vi "Main.vi"() -> ()   [LabVIEW 2016]
uses:
  Code/MainFGV/FGV_mods.ctl
  Code/TypeDefs/specimen_info.ctl
  <vilib>/Analysis/baseanly.llb/Mean (DBL).vi
  <vilib>/Analysis/NI_AALBase.lvlib
panel:
  out "Resultados":string[][](table)
  out "plot":cluster{"strain":dbl[], "stress":dbl[]}[](graph) caption="XY Graph"
  in  "test_file":path caption="Arquivo do ensaio"
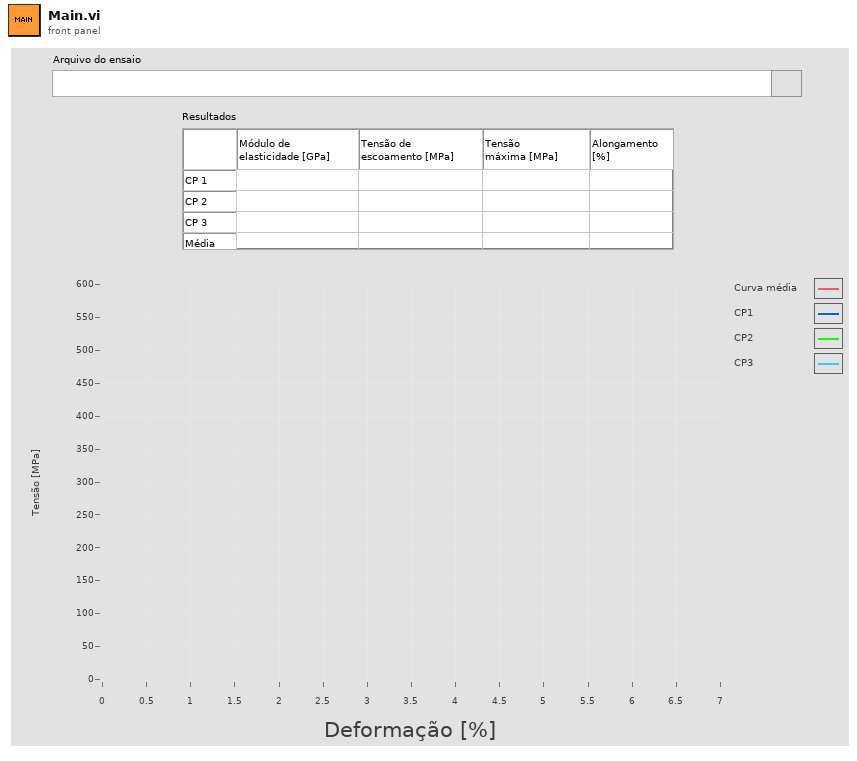
[diagram p1: front panel]
types:
  T1 = typedef "specimen_info.ctl" = cluster{"E":dbl, "Sy":dbl, "Sut":dbl, "eps max":dbl}
  T2 = typedef "FGV_mods.ctl" = enum16{"Init", "read_headers", "read_file", "plot", "process", "End"}
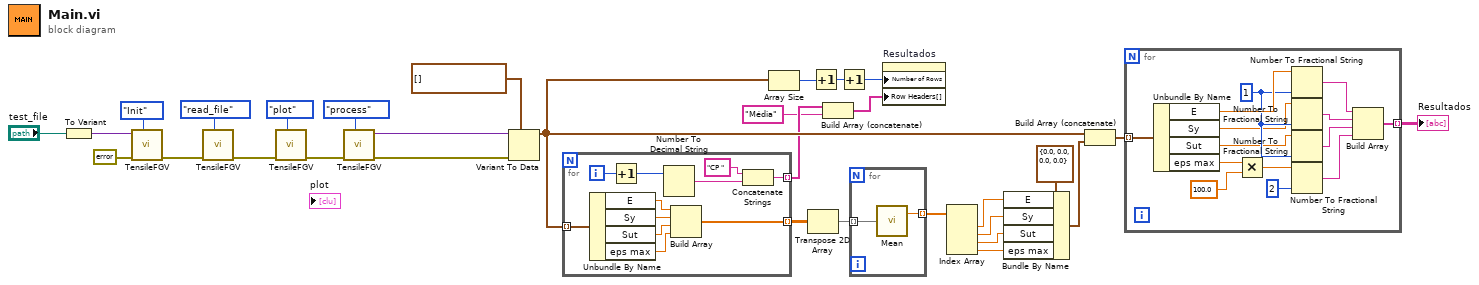
[diagram p0: block diagram]
diagram:
  n1 = To Variant(anything="test_file") -> (Variant=w31:variant)
  n2 = call "TensileFGV.vi"("FGV_mods"=FGV_mods."Init", "Error In"=errorcluster {"status"=FALSE, "code"=0, "source"=""}, "DataIn"=w31) -> ("Error Out"=w27:errorcluster)  [unwired: 7 in, 1 out]
  n3 = call "TensileFGV.vi"("FGV_mods"=FGV_mods."read_file", "Error In"=w27) -> ("Error Out"=w24:errorcluster)  [unwired: 8 in, 1 out]
  n4 = call "TensileFGV.vi"("FGV_mods"=FGV_mods."plot", "Error In"=w24) -> ("Error Out"=w22:errorcluster)  [unwired: 8 in, 1 out]
  n5 = call "TensileFGV.vi"("FGV_mods"=FGV_mods."process", "Error In"=w22) -> ("Error Out"=w21:errorcluster, "DataOut"=w20:variant)  [unwired: 8 in]
  n6 = Variant To Data(error in=w21, type=T1[] [] ("specimen_info"), Variant=w20) -> (data=w7:T1[])  [unwired: 1 out]
  n7 = for {
    tunnel: w7 -> [w42] mode=indexing
    tunnel: [w37] -> w17 mode=indexing
    tunnel: [w32] -> w3 mode=indexing
    i -> [w36]
    n8 = Unbundle By Name(w42) -> ("E"=w41:dbl, "Sy"=w40:dbl, "Sut"=w39:dbl, "eps max"=w38:dbl)
    n9 = Increment(x=w36) -> (x+1=w35:i32)
    n10 = Number To Decimal String(number=w35) -> (decimal integer string=w34:string)  [unwired: 1 in]
    n11 = Build Array(w41, w40, w39, w38) -> (w37:dbl[])
    n12 = Concatenate Strings("CP " ("string"), w34) -> (w32:string)
  }
  n13 = Array Size(array=w7) -> (size(s)=w6:i32)
  n14 = Transpose 2D Array(2D array=w17) -> (transposed array=w16:dbl[][])
  n15 = Increment(x=w6) -> (x+1=w5:i32)
  n16 = Build Array (concatenate)(w3, "Média" ("string")) -> (w1:string[])
  n17 = Increment(x=w5) -> (x+1=w4:i32)
  n18 = for {
    tunnel: w16 -> [w44] mode=indexing
    tunnel: [w43] -> w14 mode=indexing
    n19 = call-poly <vilib>:"Mean.vi"("X"=w44) -> ("mean"=w43:dbl)  [unwired: 1 out]
  }
  n20 = property on="Resultados" class="Tbl (strict)"("Number of Rows"=w4, "Row Headers[]"=w1) -> ()  [unwired: 2 in, 2 out]
  n21 = Index Array(array=w14) -> (element #1=w13:dbl, element #2=w12:dbl, element #3=w11:dbl, element #4=w10:dbl)  [unwired: 4 in]
  n22 = Bundle By Name(cluster=T1 {"E"=0.0, "Sy"=0.0, "Sut"=0.0, "eps max"=0.0} ("specimen_info"), "E"=w13, "Sy"=w12, "Sut"=w11, "eps max"=w10) -> (w9:T1)
  n23 = Build Array (concatenate)(w7, w9) -> (w8:T1[])
  n24 = for {
    tunnel: w8 -> [w58] mode=indexing
    tunnel: [w55] -> w18 mode=indexing
    w50 = i16 1 ("precision (6)")
    n25 = Unbundle By Name(w58) -> ("E"=w51:dbl, "Sy"=w49:dbl, "Sut"=w48:dbl, "eps max"=w57:dbl)
    n26 = Multiply(x=w57, y=100.0) -> (x*y=w53:dbl)
    n27 = Number To Fractional String(number=w51, precision (6)=w50) -> (F-format string=w45:string)  [unwired: 2 in]
    n28 = Number To Fractional String(number=w49, precision (6)=w50) -> (F-format string=w46:string)  [unwired: 2 in]
    n29 = Number To Fractional String(number=w48, precision (6)=w50) -> (F-format string=w47:string)  [unwired: 2 in]
    n30 = Number To Fractional String(number=w53, precision (6)=i16 2) -> (F-format string=w52:string)  [unwired: 2 in]
    n31 = Build Array(w45, w46, w47, w52) -> (w55:string[])
  }
  "Resultados" <- w18
